vi "Release and Unregister.vi"(10 "Actor":refnum<class "Actor.lvclass">) -> (2 "Unhandled Msgs":refnum<class "Msg.lvclass">[](array[class]))   [LabVIEW 2025, in "jettl.lvlib" / "Actor.lvlib"]
uses:
  Actor.lvlib
  Actor/Actor.lvclass
  Msg/Msg.lvclass
  Attributes/Attributes/Attributes.lvclass
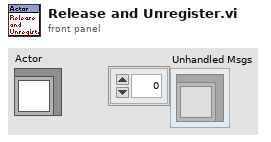
[diagram p1: front panel]
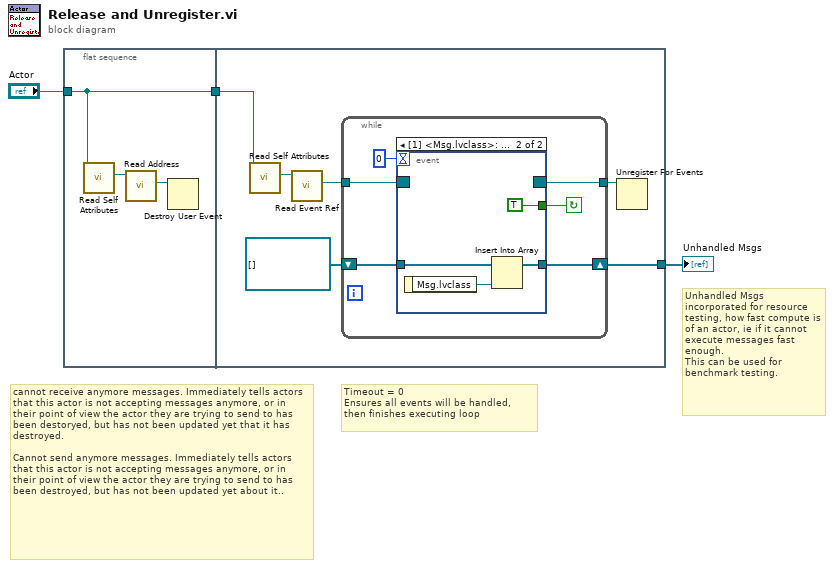
[diagram p0: block diagram]
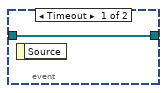
[diagram p2: hidden frame]
diagram:
  # "Unhandled Msgs incorporated for resource testing, how fast compute is of an actor, ie if it cannot execute messages fast enough.\nThis can be used for benchmark testing."
  # "Timeout = 0\nEnsures all events will be handled, then finishes executing loop"
  # "cannot receive anymore messages. Immediately tells actors that this actor is not accepting messages anymore, or in their point of view the actor they are trying to send to has been destoryed, but has not been updated yet that it has destroyed.\n\nCannot send anymore messages. Immediately tells actors that this actor is not accepting messages anymore, or in their point of view the actor they are trying to send to has been destroyed, but has not been updated yet about it.."
  n1 = flat-sequence {
    tunnel: "Actor" -> [w4]
    tunnel: [w4] -> w1
    tunnel: w1 -> [w8]
    tunnel: [w9] -> w3
    frame #0 {
      n2 = call-dynamic "Read Self Attributes.vi"("Actor in"=w4) -> ("Self Attributes"=w6:refnum<class "Attributes.lvclass">)  [unwired: 10 in]
      n3 = call-dynamic "Read Address.vi"("Attributes in"=w6) -> ("Address"=w5:refnum<user-event>)  [unwired: 10 in]
      n4 = Destroy User Event(user event=w5) -> ()  [unwired: 1 in, 1 out]
    }
    frame #1 {
      n5 = call-dynamic "Read Self Attributes.vi"("Actor in"=w8) -> ("Self Attributes"=w12:refnum<class "Attributes.lvclass">)  [unwired: 10 in]
      n6 = call-dynamic "Read Event Ref.vi"("Attributes in"=w12) -> ("Event Ref"=w10:refnum<event-registration>)  [unwired: 10 in]
      n7 = while {
        shift-right: [w17] -> w9
        shift-left: refnum<class "Msg.lvclass">[] [] -> [w18]
        tunnel: w10 -> [w16]
        tunnel: [w13] -> w7
        stop <- w15 continue-if-true
        n8 = event shown="[1] <Msg.lvclass>: User Event" {
          selector: w16 -> [_ _]
          dyn-events: [_ _] -> w13
          timeout: 0 -> [_ _]
          tunnel: w18 -> [w19 w23]
          tunnel: [w19 w22] -> w17
          tunnel: [_ TRUE] -> w15
          event Timeout {
            n9 = event-data() -> ()  [unwired: 1 in, 1 out]
          }
          event User Event {
            n10 = event-data() -> ("Msg.lvclass"=w21:refnum<class "Msg.lvclass">)  [unwired: 1 in]
            n11 = Insert Into Array(array=w23, new element=w21) -> (w22:refnum<class "Msg.lvclass">[])  [unwired: 1 in]
          }
        }
      }
      n12 = Unregister For Events(event registration refnum=w7) -> ()  [unwired: 1 in, 1 out]
    }
  }
  "Unhandled Msgs" <- w3
